vi "Current Value.vi"(8 "error in (no error)":errorcluster, 11 "StringChannel in":refnum<class "StringChannel.lvclass">) -> (0 "error out":errorcluster, 1 "Timestamp":dbl, 2 "String":string, 3 "StringChannel out":refnum<class "StringChannel.lvclass">)   [LabVIEW 2020, in "Vecto.lvlib" / "StringChannel.lvclass"]
uses:
  StringChannel.lvclass
  StringChannel.lvclass/StringChannel.ctl
  StringGroup/StringGroup.lvclass
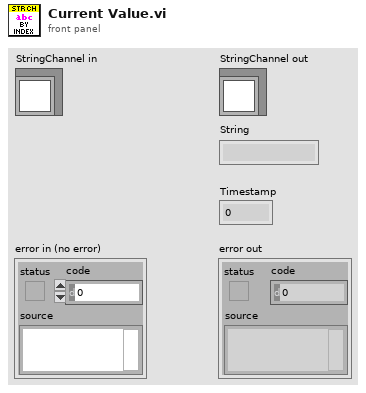
[diagram p1: front panel]
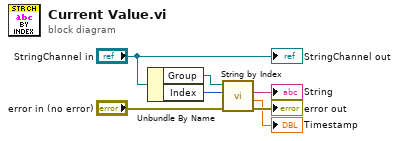
[diagram p0: block diagram]
diagram:
  n1 = Unbundle By Name("StringChannel in") -> ("Group"=w6:refnum<class "StringGroup.lvclass">, "Index"=w5:i32)
  n2 = call "String by Index.vi"("error in (no error)"="error in (no error)", "Index"=w5, "StringGroup in"=w6) -> ("error out"=→"error out":errorcluster, "Timestamp"=→"Timestamp":dbl, "String"=→"String":string)  [unwired: 5 in, 1 out]
  "StringChannel out" <- "StringChannel in"
